vi "Sliders Teleop (PC).vi"() -> ()   [LabVIEW 2013]
uses:
  labview_ros/sensor_msgs/JointState.ctl
  labview_ros/std_msgs/Header.ctl
  Telemanipulation/Helpers/Helpers.lvlib
panel:
  out "UDP Receiver":cluster{"Rate (Hz)":dbl, "Status":errorcluster}
  in  "stop":bool
  in  "Joint Names":string[](array[string])=["SA", "SE", "EL", "WP", "WY", "WR"]
  in  "PXI":T1={"IP"="192.168.0.4", "Read Port"=5052, "Write Port"=5051}
  out "UDP Sender":cluster{"Rate (Hz)":dbl, "Status":errorcluster}
  in  "WR":dbl(slide)=-0.9473827382931216 scale=-3.14..3.14
  in  "WY":dbl(slide)=0.3565705572681916 scale=-0.7..1.2
  in  "WP":dbl(slide)=-0.29450757439331093 scale=-0.7..1.2
  in  "EL":dbl(slide)=3.229844911017393 scale=-1.0..2.1
  in  "SE":dbl(slide)=-1.3453457540222367 scale=-1.58..0.53
  in  "SA":dbl(slide)=0.31900452488687786 scale=-1.58..1.58
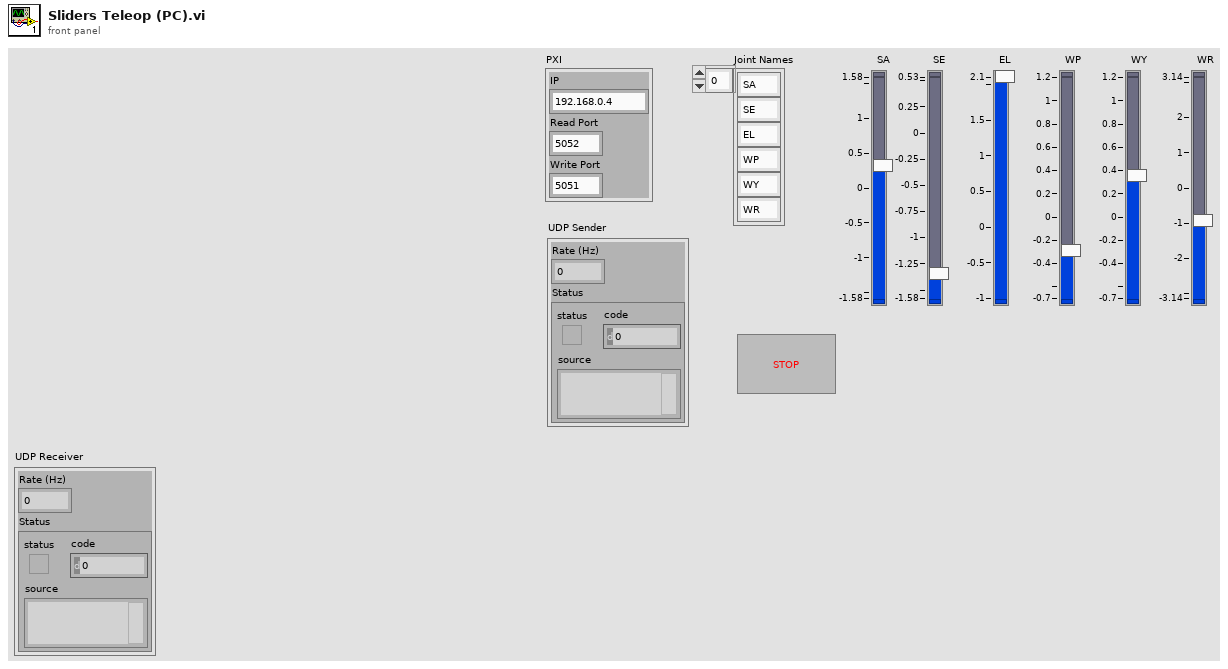
[diagram p1: front panel]
types:
  T1 = cluster{"IP":string, "Read Port":u16, "Write Port":u16}
  T2 = enum16{"big-endian, network order", "native, host order", "little-endian"}
  T3 = typedef "JointState.ctl" = cluster{"header":T4, "name":string[], "position":dbl[], "velocity":dbl[], "effort":dbl[]}
  T4 = typedef "Header.ctl" = cluster{"seq":u32, "stamp":cluster{"sec":i32, "nsec":i32}, "frame_id":string}
  T5 = cluster{"seq":u32, "stamp":cluster{"sec":i32, "nsec":i32}, "frame_id":string}
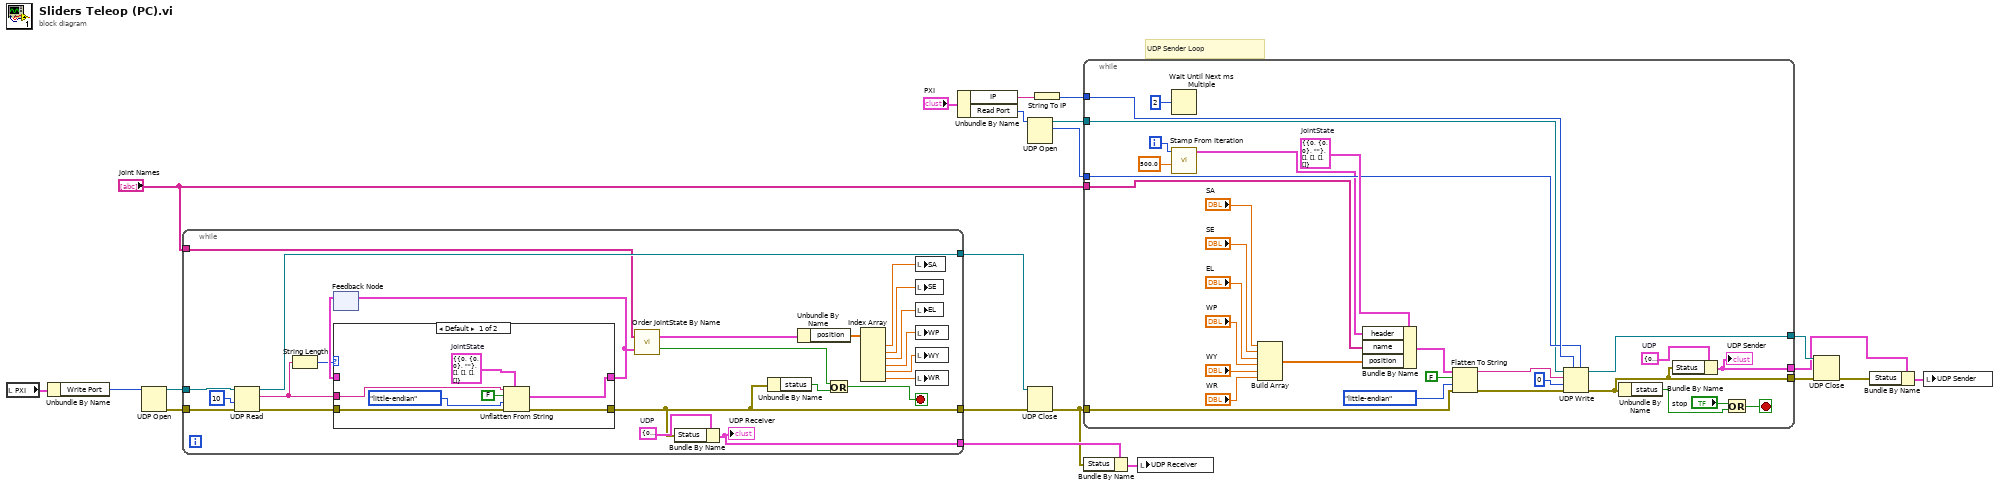
[diagram p0: block diagram]
diagram:
  # "UDP Sender Loop"
  n1 = local read "PXI"() -> (w4:T1)
  n2 = Unbundle By Name(w4) -> ("Write Port"=w3:u16)
  n3 = UDP Open(11:w3) -> (port=w1:refnum<k16>, 0:w5:errorcluster)  [unwired: 1 in, 4 out]
  n4 = while {
    tunnel: [w25] -> w6
    tunnel: [w45] -> w7
    tunnel: "Joint Names" -> [w42]
    tunnel: [w39] -> w9
    tunnel: w5 -> [w35]
    tunnel: w1 -> [w27]
    stop <- w22 stop-if-true
    w40 = cluster{"Rate (Hz)":dbl, "Status":errorcluster} {"Rate (Hz)"=0.0, "Status"={"status"=FALSE, "code"=0, "source"=""}}  # UDP
    n5 = UDP Read(connection ID=w27, timeout ms (25000)=10 ("timeout (ms)"), 8:w35) -> (data out=w44:string, error out=w26:errorcluster, 3:w45:refnum<k16>)  [unwired: 1 in, 2 out]
    n6 = String Length(string=w44) -> (length=w36:i32)
    n7 = feedback #1() -> (w38:T3)  [unwired: 1 in]
    n8 = case shown="Default" w36 {
      tunnel: w44 -> [w51 _]
      tunnel: w26 -> [w50 w54]
      tunnel: [w49 w54] -> w25
      tunnel: [w47 w53] -> w37
      tunnel: w38 -> [_ w53]
      frame Default {
        w46 = T3 {"header"={"seq"=0, "stamp"={"sec"=0, "nsec"=0}, "frame_id"=""}, "name"=[], "position"=[], "velocity"=[], "effort"=[]}  # JointState
        n9 = Unflatten From String(type=w46, binary string=w51, data includes array or string size? (T)=FALSE, byte order (0:big-endian, network order)=T2."little-endian", error in (no error)=w50) -> (value=w47:T3, error out=w49:errorcluster)  [unwired: 1 out]
      }
      frame 0 {
      }
    }
    n10 = feedback-in #1(w37) -> ()
    n11 = call "Order JointState By Name.vi"("JointState In"=w37, "Ordered Joint Names"=w42) -> ("all found?"=w23:bool, "JointState Out"=w41:T3)
    n12 = Bundle By Name(cluster=w40, "Status"=w25) -> (w39:cluster{"Rate (Hz)":dbl, "Status":errorcluster})
    "UDP Receiver" <- w39
    n13 = Unbundle By Name(w25) -> ("status"=w24:bool)
    n14 = Unbundle By Name(w41) -> ("position"=w34:dbl[])
    n15 = Or(x=w23, y=w24) -> (x .or. y?=w22:bool)
    n16 = Index Array(array=w34) -> (element #1=w33:dbl, element #2=w32:dbl, element #3=w31:dbl, element #4=w30:dbl, element #5=w29:dbl, element #6=w28:dbl)  [unwired: 6 in]
    n17 = local write "SA"(w33) -> ()
    n18 = local write "SE"(w32) -> ()
    n19 = local write "EL"(w31) -> ()
    n20 = local write "WP"(w30) -> ()
    n21 = local write "WY"(w29) -> ()
    n22 = local write "WR"(w28) -> ()
  }
  n23 = Unbundle By Name("PXI") -> ("IP"=w20:string, "Read Port"=w15:u16)
  n24 = UDP Open(11:w15) -> (port=w17:refnum<k16>, 2:w18:u16)  [unwired: 1 in, 4 out]
  n25 = UDP Close(connection ID=w7, 8:w6) -> (error out=w2:errorcluster)  [unwired: 1 out]
  n26 = String To IP(1:w20) -> (0:w19:u32)
  n27 = while {
    tunnel: [w67] -> w14
    tunnel: "Joint Names" -> [w83]
    tunnel: w19 -> [w78]
    tunnel: w18 -> [w77]
    tunnel: w17 -> [w76]
    tunnel: [w74] -> w16
    tunnel: [w66] -> w11
    tunnel: w2 -> [w55]
    i -> [w73]
    stop <- w56 stop-if-true
    w68 = cluster{"Rate (Hz)":dbl, "Status":errorcluster} {"Rate (Hz)"=0.0, "Status"={"status"=FALSE, "code"=0, "source"=""}}  # UDP
    w82 = T3 {"header"={"seq"=0, "stamp"={"sec"=0, "nsec"=0}, "frame_id"=""}, "name"=[], "position"=[], "velocity"=[], "effort"=[]}  # JointState
    n28 = Wait Until Next ms Multiple(millisecond multiple=u32 2) -> ()  [unwired: 1 out]
    n29 = call "Stamp From Iteration.vi"("Rate (Hz)"=500.0, "Iteration"=w73) -> ("Header"=w71:T5)  [unwired: 9 in]
    n30 = Build Array("SA", "SE", "EL", "WP", "WY", "WR") -> (w58:dbl[])
    n31 = Bundle By Name(cluster=w82, "header"=w71, "name"=w83, "position"=w58) -> (w84:T3)
    n32 = Flatten To String(anything=w84, prepend array or string size? (T)=FALSE, byte order (0:big-endian, network order)=T2."little-endian", error in (no error)=w55) -> (data string=w81:string, error out=w75:errorcluster)  [unwired: 1 out]
    n33 = UDP Write(address=w78, port or service name=w77, connection ID=w76, data in=w81, 8:w75, 9:0 ("timeout ms (25000)")) -> (error out=w67:errorcluster, 3:w74:refnum<k16>)
    n34 = Unbundle By Name(w67) -> ("status"=w69:bool)
    n35 = Bundle By Name(cluster=w68, "Status"=w67) -> (w66:cluster{"Rate (Hz)":dbl, "Status":errorcluster})
    "UDP Sender" <- w66
    n36 = Or(x="stop", y=w69) -> (x .or. y?=w56:bool)
  }
  n37 = Bundle By Name(cluster=w9, "Status"=w2) -> (w8:cluster{"Rate (Hz)":dbl, "Status":errorcluster})
  n38 = local write "UDP Receiver"(w8) -> ()
  n39 = UDP Close(connection ID=w16, 8:w14) -> (error out=w13:errorcluster)  [unwired: 1 out]
  n40 = Bundle By Name(cluster=w11, "Status"=w13) -> (w12:cluster{"Rate (Hz)":dbl, "Status":errorcluster})
  n41 = local write "UDP Sender"(w12) -> ()
